vi "H036 Harsh Pandit SCADA Lab 6c Sem 6.vi"() -> ()   [LabVIEW 2018]
uses:
  <vilib>/Analysis/baseanly.llb/Real Determinant.vi
  <vilib>/Analysis/NI_AALBase.lvlib
panel:
  out "determinant":dbl format="%.2e"
  out "Array Display":dbl[][](array[numeric])
  in  "Array":dbl[][](array[numeric])
  # "Experiment 6c: Create a VI to form 2 dimensional array of 5 x 5 elements. Also find determinent \nof 2 by 2 matrix"
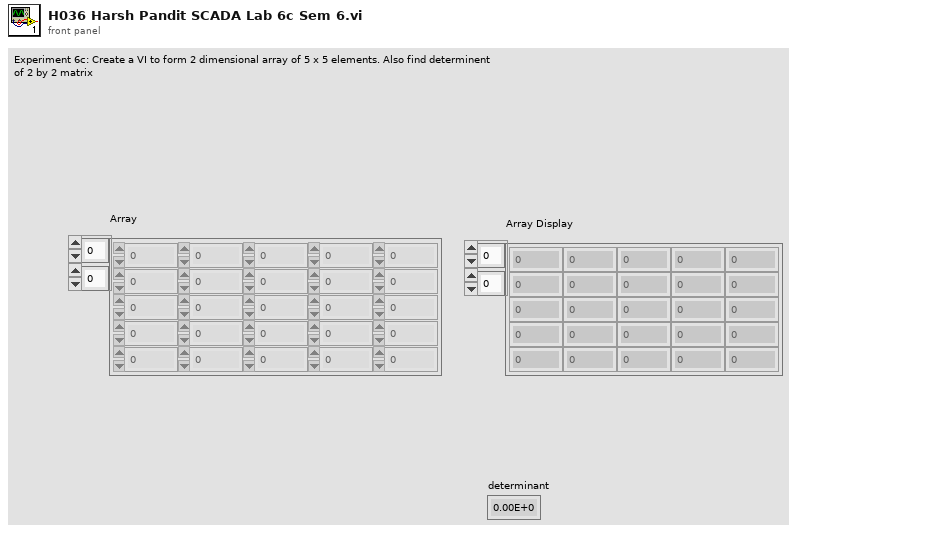
[diagram p1: front panel]
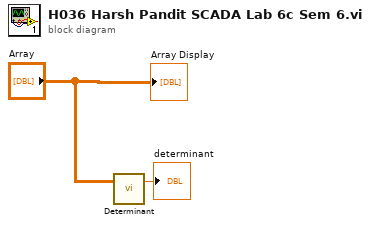
[diagram p0: block diagram]
diagram:
  n1 = call-poly <vilib>:"Determinant.vi"("Input Matrix"="Array") -> ("determinant"=→"determinant":dbl)  [unwired: 1 in, 1 out]
  "Array Display" <- "Array"
